vi "Seeder Control.vi"(7 "Mode":bool, 9 "Duty Cycle (%)":dbl=4.0, 11 "Seed Pulse (s)":dbl=10.0 min=3.0) -> (2 "Seeder On":bool, 3 "Cycle Length (s)":dbl=8.0)   [LabVIEW 2014]
uses:
  <vilib>/Platform/TimedLoop/XDataNode/nitl_modes.ctl
  <vilib>/Platform/TimedLoop/XDataNode/timing_clust.ctl
  <vilib>/Platform/TimedLoop/XDataNode/wakeup.ctl
  <vilib>/Platform/TimedLoop/XDataNode/XDataNode.xnode
  <vilib>/Platform/TimedLoop/XDataNode/XDNodeRunTimeDep.lvlib
panel:
  out "Next Seed":dbl(slide) scale=0.0..1.0
  in  "Stop Button":bool
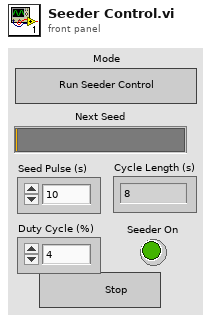
[diagram p1: front panel]
types:
  T1 = typedef "XDNodeRunTimeDep.lvlib/nitl_modes.ctl" = enum32{"No Change", "Process missed periods, maintain original phase", "Discard missed periods, maintain original phase", "Process missed periods, ignore original phase", "Discard missed periods, ignore original phase"}
  T2 = typedef "XDNodeRunTimeDep.lvlib/timing_clust.ctl" = cluster{"Expected End [f-1]":u64, "Actual End [f-1]":u64, "Finished Late? [f-1]":bool, "Expected End [i-1]":u64, "Actual End [i-1]":u64, "Finished Late? [i-1]":bool, "Expected Start [i]":u64, "Actual Start [i]":u64, "Expected Start [f]":u64, "Actual Start [f]":u64, "Source Name":string, "Structure Name":string, "Period":i64, "Deadline":i64, "Offset":i64, "Start":i64, "Priority":i32, "Timeout":i32, "Mode":T1, "Wakeup Reason":T3, "Error":errorcluster, "Source Type":string, "Secondary Source Type":string, "Global End Time":u64, "Global Start Time":u64, "Frame Duration":u64, "Iteration Duration":u64, "Assigned CPU":i32, "I/O Scan Engine Mode":u32}
  T3 = typedef "XDNodeRunTimeDep.lvlib/wakeup.ctl" = enum32{"Normal", "Aborted", "Asynchronous wakeup", "Timing source error", "Timed loop error", "Timeout"}
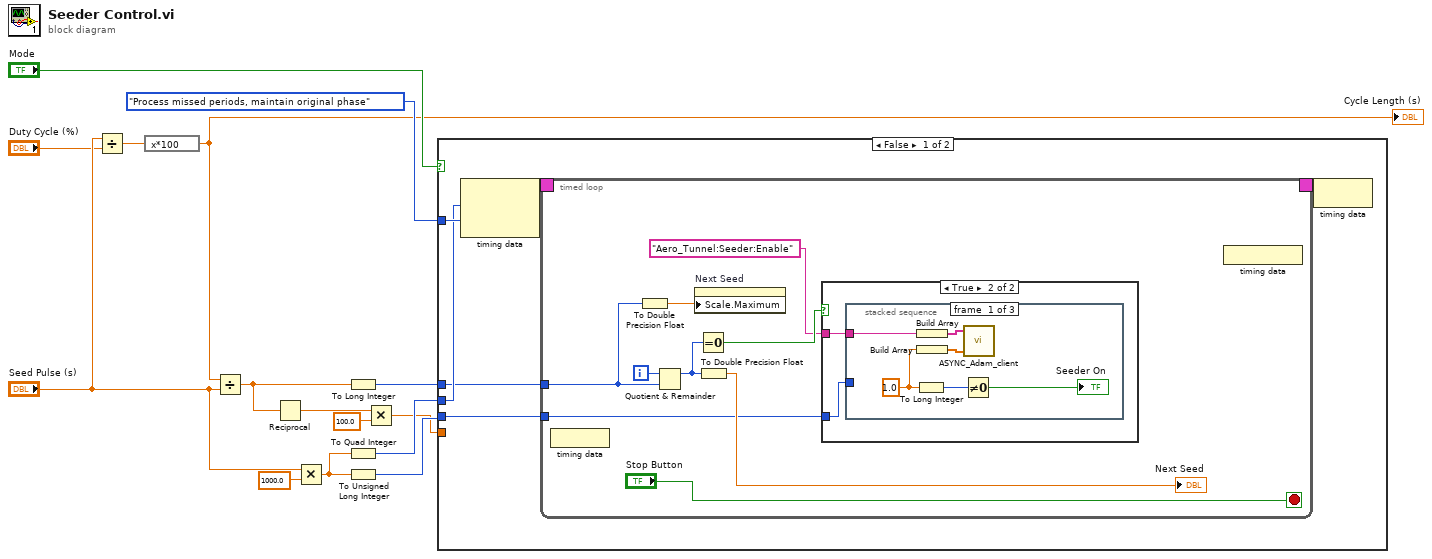
[diagram p0: block diagram]
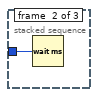
[diagram p3: hidden frame]
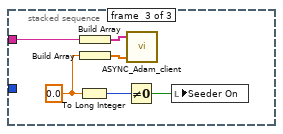
[diagram p4: hidden frame]
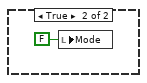
[diagram p5: hidden frame]
diagram:
  n1 = Divide(x="Seed Pulse (s)", y="Duty Cycle (%)") -> (x/y=w2:dbl)
  n2 = expression code="x*100"(w2) -> (w1:dbl)
  "Cycle Length (s)" <- w1
  n3 = Divide(x=w1, y="Seed Pulse (s)") -> (x/y=w7:dbl)
  n4 = Reciprocal(x=w7) -> (1/x=w6:dbl)
  n5 = Multiply(x="Seed Pulse (s)", y=1000.0) -> (x*y=w12:dbl)
  n6 = To Long Integer(number=w7) -> (32bit integer=w10:i32)
  n7 = To Quad Integer(1:w12) -> (0:w13:i64)
  n8 = To Unsigned Long Integer(number=w12) -> (unsigned 32bit integer=w11:u32)
  n9 = Multiply(x=w6, y=100.0) -> (x*y=w5:dbl)
  n10 = case shown="False" "Mode" {
    tunnel: nitl_modes."Process missed periods, maintain original phase" ("Mode") -> [w19 _]
    tunnel: w13 -> [w18 _]
    tunnel: w11 -> [w17 _]
    tunnel: w10 -> [w16 _]
    tunnel: w5 -> [_ _]
    frame False {
      n11 = node-c288(w18, w19) -> (w21:T2)
      n12 = timed-loop {
        timing: w21 -> [_]
        timing-out: [_] -> w20
        tunnel: w17 -> [w23]
        tunnel: w16 -> [w22]
        i -> [w29]
        stop <- "Stop Button" stop-if-true
        n13 = node-c288() -> ()  [unwired: 1 in]
        n14 = To Double Precision Float(number=w22) -> (double precision float=w26:dbl)
        n15 = Quotient & Remainder(x=w29, y=w22) -> (x-y*floor(x/y)=w24:i32)  [unwired: 1 out]
        n16 = property on="Next Seed" class="Slide (strict)"("Scale.Maximum"=w26) -> ()  [unwired: 2 in, 2 out]
        n17 = Equal To 0?(x=w24) -> (x = 0?=w28:bool)
        n18 = To Double Precision Float(number=w24) -> (double precision float=→"Next Seed":dbl)
        n19 = case shown="True" w28 {
          tunnel: "Aero_Tunnel:Seeder:Enable" -> [_ w32]
          tunnel: w23 -> [_ w31]
          frame False {
          }
          frame True {
            n20 = stacked-sequence {
              tunnel: w32 -> [w33 _ w41]
              tunnel: w31 -> [_ w39 _]
              frame #0 {
                w34 = 1.0 ("New Value")
                n21 = To Long Integer(number=w34) -> (32bit integer=w38:i32)
                n22 = Build Array(w33) -> (w35:string[])
                n23 = Build Array(w34) -> (w36:dbl[])
                n24 = Not Equal To 0?(x=w38) -> (x != 0?=→"Seeder On":bool)
                n25 = call "ASYNC_Adam_client.vi"("Values"=w36, "Channel Names"=w35) -> ()  [unwired: 1 in, 2 out]
              }
              frame #1 {
                n26 = Wait (ms)(milliseconds to wait=w39) -> ()  [unwired: 1 out]
              }
              frame #2 {
                w40 = 0.0 ("New Value")
                n27 = To Long Integer(number=w40) -> (32bit integer=w45:i32)
                n28 = Build Array(w41) -> (w42:string[])
                n29 = Build Array(w40) -> (w43:dbl[])
                n30 = Not Equal To 0?(x=w45) -> (x != 0?=w44:bool)
                n31 = call "ASYNC_Adam_client.vi"("Values"=w43, "Channel Names"=w42) -> ()  [unwired: 1 in, 2 out]
                n32 = local write "Seeder On"(w44) -> ()
              }
            }
          }
        }
        n33 = node-c288() -> ()  [unwired: 1 out]
      }
      n34 = node-c288(w20) -> ()
    }
    frame True {
      n35 = local write "Mode"(FALSE ("Mode")) -> ()
    }
  }
